vi "Update Single Light.vi"(8 "error in (no error)":errorcluster, 9 "Values":T2[](array[typedef]), 10 "Light Selection":T1, 11 "LightsPanel in":refnum<class "LightsPanel.lvclass">) -> (0 "error out":errorcluster, 3 "LightsPanel out":refnum<class "LightsPanel.lvclass">)   [LabVIEW 2022 SP3, in "TouchControl.lvlib" / "LightsPanel.lvclass"]
uses:
  LightsPanel.lvclass
  Update Status.ctl
  Light Selection.ctl
  Update Type.ctl
  LightsPanel.lvclass/LightsPanel.ctl
  TouchControl.lvlib
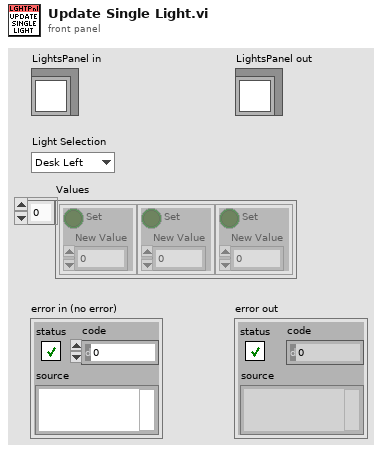
[diagram p1: front panel]
types:
  T1 = typedef "TouchControl.lvlib/Light Selection.ctl" = enum16{"Desk Left", "Desk Right", "Printer"}
  T2 = typedef "TouchControl.lvlib/LightsPanel.lvclass/Update Status.ctl" = cluster{"Set":bool, "New Value":dbl}
  T3 = typedef "TouchControl.lvlib/LightsPanel.lvclass/Update Type.ctl" = enum16{"Light On", "Temp", "Brightness"}
  T4 = typedef "TouchControl.lvlib/Light Config.ctl" = cluster{"Desk Left":string, "Desk Right":string, "Printer":string}
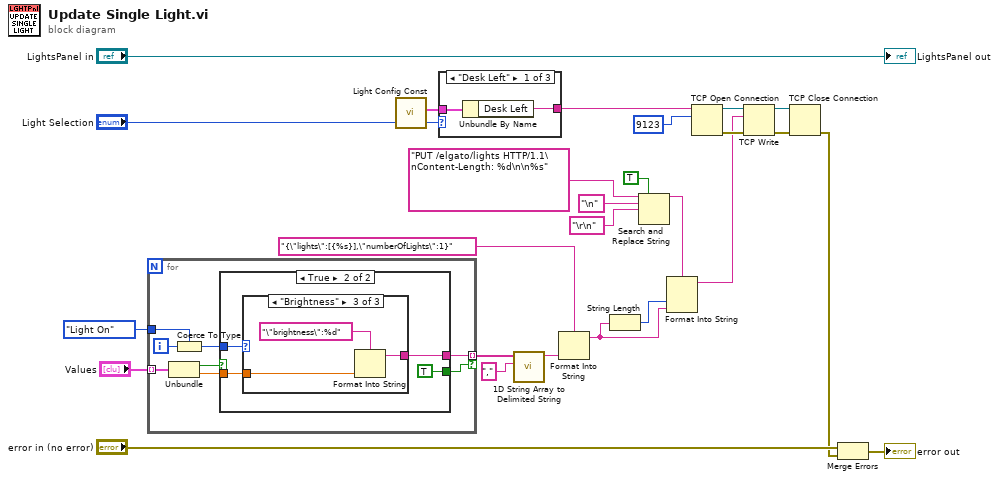
[diagram p0: block diagram]
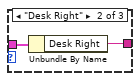
[diagram p2: hidden frame]
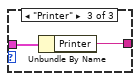
[diagram p3: hidden frame]
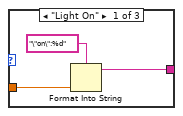
[diagram p5: hidden frame]
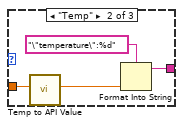
[diagram p6: hidden frame]
diagram:
  n1 = for {
    tunnel: "Values" -> [w32] mode=indexing
    tunnel: Update_Type."Light On" ("Update Type") -> [w33]
    tunnel: [w28] -> w22 mode=indexing if=w27
    i -> [w34]
    n2 = Unbundle(w32) -> ("Set"=w31:bool, "New Value"=w29:dbl)
    n3 = Coerce To Type(0:w34, 1:w33) -> (2:w30:T3)
    n4 = case shown="True" w31 {
      tunnel: w30 -> [_ w38]
      tunnel: w29 -> [_ w37]
      tunnel: [_ w36] -> w28
      tunnel: [_ TRUE] -> w27
      frame False {
      }
      frame True {
        n5 = case shown="\"Brightness\"" w38 {
          tunnel: w37 -> [w41 w45 w48]
          tunnel: [w39 w42 w46] -> w36
          frame "Light On" {
            n6 = Format Into String(format string="\"on\":%d", w41) -> (resulting string=w39:string)  [unwired: 2 in, 1 out]
          }
          frame "Temp" {
            n7 = call "Temp to API Value.vi"("Color Temp"=w45) -> ("API Temp"=w44:dbl)  [unwired: 10 in]
            n8 = Format Into String(format string="\"temperature\":%d", w44) -> (resulting string=w42:string)  [unwired: 2 in, 1 out]
          }
          frame "Brightness" {
            n9 = Format Into String(format string="\"brightness\":%d", w48) -> (resulting string=w46:string)  [unwired: 2 in, 1 out]
          }
        }
      }
    }
  }
  n10 = call "Light Config Const.vi"() -> ("Light Config"=w8:T4)  [unwired: 11 in]
  n11 = case shown="\"Desk Left\"" "Light Selection" {
    tunnel: w8 -> [w50 w52 w54]
    tunnel: [w49 w51 w53] -> w6
    frame "Desk Left" {
      n12 = Unbundle By Name(w50) -> ("Desk Left"=w49:string)
    }
    frame "Desk Right" {
      n13 = Unbundle By Name(w52) -> ("Desk Right"=w51:string)
    }
    frame "Printer" {
      n14 = Unbundle By Name(w54) -> ("Printer"=w53:string)
    }
  }
  n15 = call <vilib>:"1D String Array to Delimited String.vi"("delimiter"=",", "string array"=w22) -> ("delimited string"=w20:string)  [unwired: 9 in]
  n16 = Format Into String(format string="{\"lights\":[{%s}],\"numberOfLights\":1}", w20) -> (resulting string=w13:string)  [unwired: 2 in, 1 out]
  n17 = String Length(string=w13) -> (length=w14:i32)
  n18 = Search and Replace String(replace all?=TRUE ("replace all? (F)"), input string="PUT /elgato/lights HTTP/1.1\nContent-Length: %d\n\n%s", search string="\n", replace string="\r\n" ("search string")) -> (result string=w12:string)  [unwired: 4 in, 3 out]
  n19 = Format Into String(format string=w12, w14, w13) -> (resulting string=w5:string)  [unwired: 2 in, 1 out]
  n20 = TCP Open Connection(address=w6, remote port or service name=u16 9123) -> (connection ID=w4:refnum<k5>, error out=w10:errorcluster)  [unwired: 3 in]
  n21 = TCP Write(connection ID=w4, data in=w5, error in (no error)=w10) -> (connection ID out=w3:refnum<k5>, error out=w9:errorcluster)  [unwired: 1 in, 1 out]
  n22 = TCP Close Connection(connection ID=w3, error in (no error)=w9) -> (error out=w1:errorcluster)  [unwired: 1 in, 1 out]
  n23 = Merge Errors("error in (no error)", w1) -> (→"error out":errorcluster)
  "LightsPanel out" <- "LightsPanel in"
